vi "FVI_Swerve_Normalise vitesses.vi"(10 "Gain":dbl=1.0, 11 "SwerveDrive in":T1) -> (3 "SwerveDrive out":T1)   [LabVIEW 2018]
uses:
  SwerveDrive.ctl
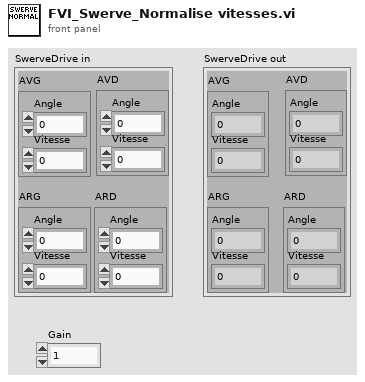
[diagram p1: front panel]
types:
  T1 = typedef "SwerveDrive.ctl" = cluster{"AVD":cluster{"Angle":dbl, "Vitesse":dbl}, "AVG":cluster{"Angle":dbl, "Vitesse":dbl}, "ARG":cluster{"Angle":dbl, "Vitesse":dbl}, "ARD":cluster{"Angle":dbl, "Vitesse":dbl}}
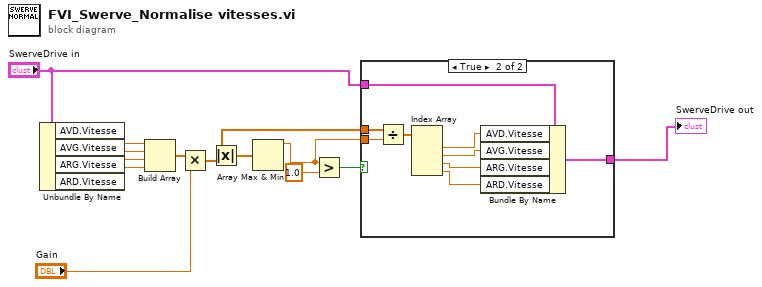
[diagram p0: block diagram]
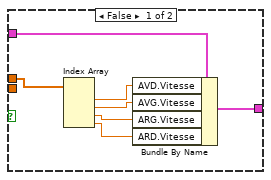
[diagram p2: hidden frame]
diagram:
  n1 = Unbundle By Name("SwerveDrive in") -> ("AVD.Vitesse"=w5:dbl, "AVG.Vitesse"=w8:dbl, "ARG.Vitesse"=w7:dbl, "ARD.Vitesse"=w6:dbl)
  n2 = Build Array(w5, w8, w7, w6) -> (w3:dbl[])
  n3 = Multiply(x=w3, y="Gain") -> (x*y=w2:dbl[])
  n4 = Absolute Value(x=w2) -> (abs(x)=w1:dbl[])
  n5 = Array Max & Min(array=w1) -> (max value=w11:dbl)  [unwired: 3 out]
  n6 = Greater?(x=w11, y=1.0) -> (0:w10:bool)
  n7 = case shown="True" w10 {
    tunnel: w2 -> [w14 w29]
    tunnel: w11 -> [_ w28]
    tunnel: "SwerveDrive in" -> [w16 w22]
    tunnel: [w15 w21] -> w13
    frame False {
      n8 = Index Array(array=w14) -> (element #1=w20:dbl, element #2=w19:dbl, element #3=w18:dbl, element #4=w17:dbl)  [unwired: 4 in]
      n9 = Bundle By Name(cluster=w16, "AVD.Vitesse"=w20, "AVG.Vitesse"=w19, "ARG.Vitesse"=w18, "ARD.Vitesse"=w17) -> (w15:T1)
    }
    frame True {
      n10 = Divide(x=w29, y=w28) -> (x/y=w27:dbl[])
      n11 = Index Array(array=w27) -> (element #1=w26:dbl, element #2=w25:dbl, element #3=w24:dbl, element #4=w23:dbl)  [unwired: 4 in]
      n12 = Bundle By Name(cluster=w22, "AVD.Vitesse"=w26, "AVG.Vitesse"=w25, "ARG.Vitesse"=w24, "ARD.Vitesse"=w23) -> (w21:T1)
    }
  }
  "SwerveDrive out" <- w13
